vi "UAS_Ground_Station_v1.02.vi"() -> ()   [LabVIEW 2020]
uses:
  <vilib>/Utility/miscctls.llb/LVForegroundBackgroundColorsTypeDef.ctl
  76567d80-d4f7-4105-a57e-45636684cd43.vi
  66f1963f-959d-441b-b800-4ec726fb55a9.vi
  2b59091c-cbc3-4e12-b608-60c3f7d5f04d.vi
  4d25b74f-ab1f-40a0-8ca1-83bd5f887b88.vi
panel:
  out "EXCEL_STATUS":string
  in  "Export":bool
  out "TimeoutCount":dbl
  out "TotalLatencyArray":dbl[](array[numeric])
  in  "Total Latency":bool
  out "Stop_buf":bool=TRUE
  in  "Rx Latency":bool
  out "RxSampleArray":dbl[](array[numeric])
  out "RxLatencyArray":dbl[](array[numeric])
  out "Rx Timer Start":dbl
  out "Latency Data":cluster{"Value":i32[], "Value":u32[]}[](graph)
  in  "Tx Latency":bool
  out "TxSampleArray":dbl[](array[numeric])
  out "TxLatencyArray":u32[](array[numeric])
  out "Rx_Index":dbl
  out "Tx_Index":dbl
  out "Tx Timer Start":u32
  in  "Tx Data":T1 {"Position(X):" format="%_6g"; "Position(Y):" format="%_6g"; "Position(Z):" format="%_6g"; "Rotation(X):" format="%_6g"; "Rotation(Y):" format="%_6g"; "Rotation(Z):" format="%_6g"; "Mode:" format="%#.6f"}
  out "Rx Data":T2
  out "number":i32
  out "Rx Struct Data":dbl[](array[numeric])
  out "Rx array":string[](array[string])
  out "Index":dbl
  out "stringBuffer":string
  out "Rx Status":bool
  out "Tx Status":bool
  in  "OK Button":bool
  out "IP":string
  out "Rx String":string
  out "Tx String":string
  in  "Rx Port":string="3000"
  in  "Tx Port":string="2390"
  in  "Address":string="192.168.1.244"
  in  "stop":bool
  # "UAS Ground Station Control"
  # "UAS UDP Latency Data"
  # "Network Configuration"
  # "Rx Data"
  # "Tx Data"
  # "Communication Controls"
  # "Status Indicators"
  # "Plot Contols"
  # "Rx"
  # "Tx"
  # "Total"
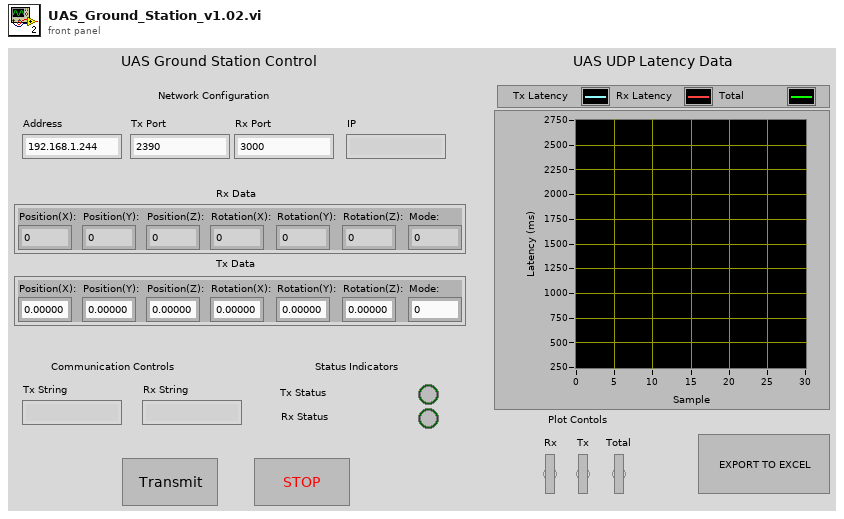
[diagram p1: front panel]
types:
  T1 = cluster{"Mode:":i32, "Rotation(Z):":dbl, "Rotation(Y):":dbl, "Rotation(X):":dbl, "Position(Z):":dbl, "Position(Y):":dbl, "Position(X):":dbl}
  T2 = cluster{"Position(X):":dbl, "Position(Y):":dbl, "Position(Z):":dbl, "Rotation(X):":dbl, "Rotation(Y):":dbl, "Rotation(Z):":dbl, "Mode:":i32}
  T3 = enum8{"Enabled", "Disabled", "Disabled and Grayed Out"}
  T4 = typedef "LVForegroundBackgroundColorsTypeDef.ctl" = cluster{"Foreground Color":u32, "Background Color":u32}
  T5 = cluster{"Value[0]":dbl, "Value[1]":dbl, "Value[2]":dbl, "Value[3]":dbl, "Value[4]":dbl, "Value[5]":dbl}
  T6 = cluster{"Value[0]":dbl, "Value[1]":dbl, "Value[2]":dbl, "Value[3]":dbl, "Value[4]":dbl, "Value[5]":dbl, "Value":i32}
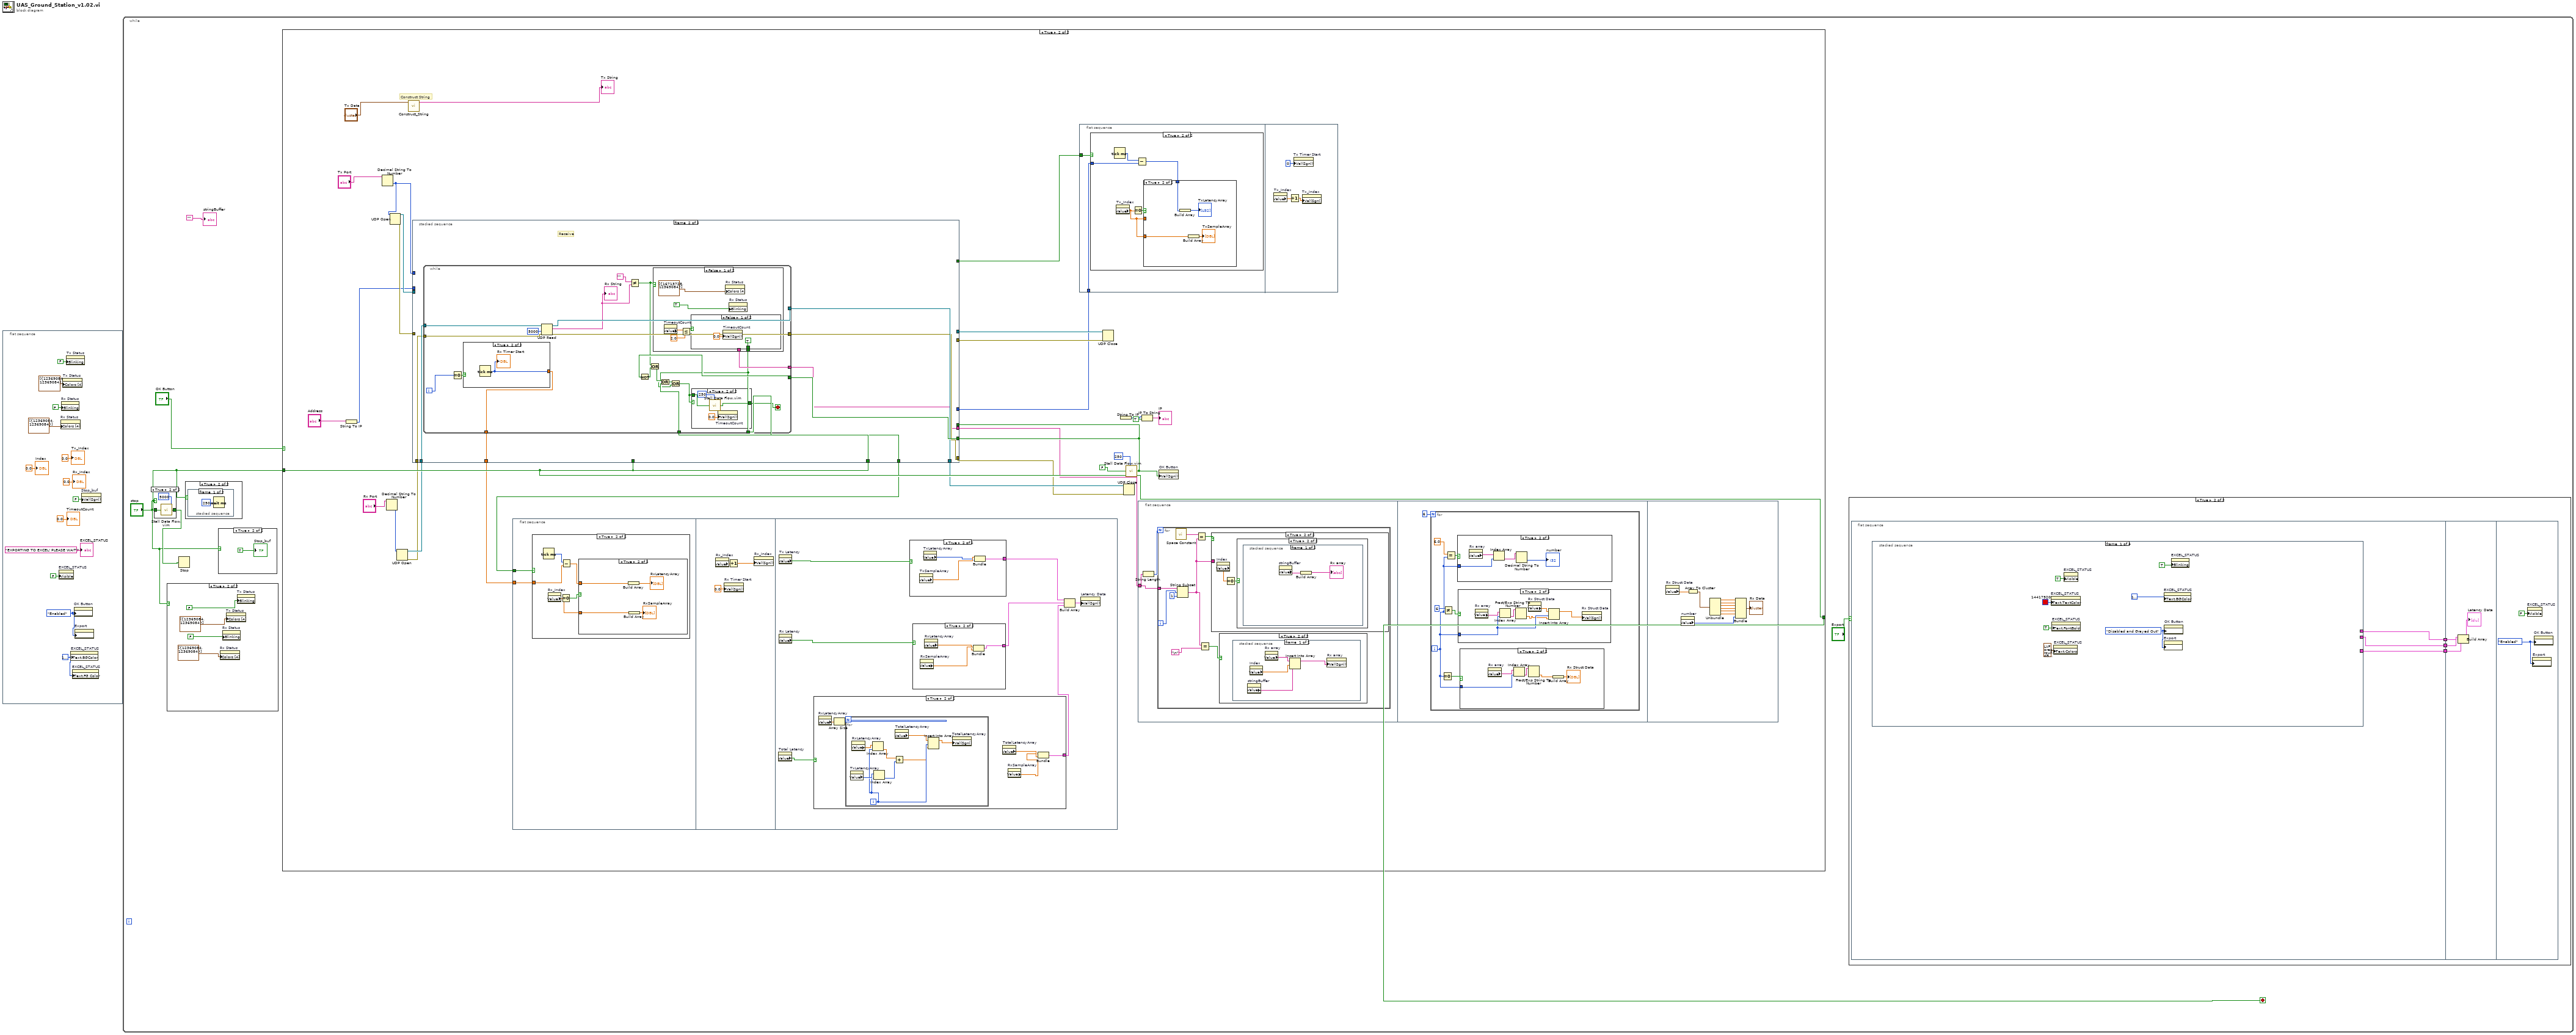
[diagram p0: block diagram]
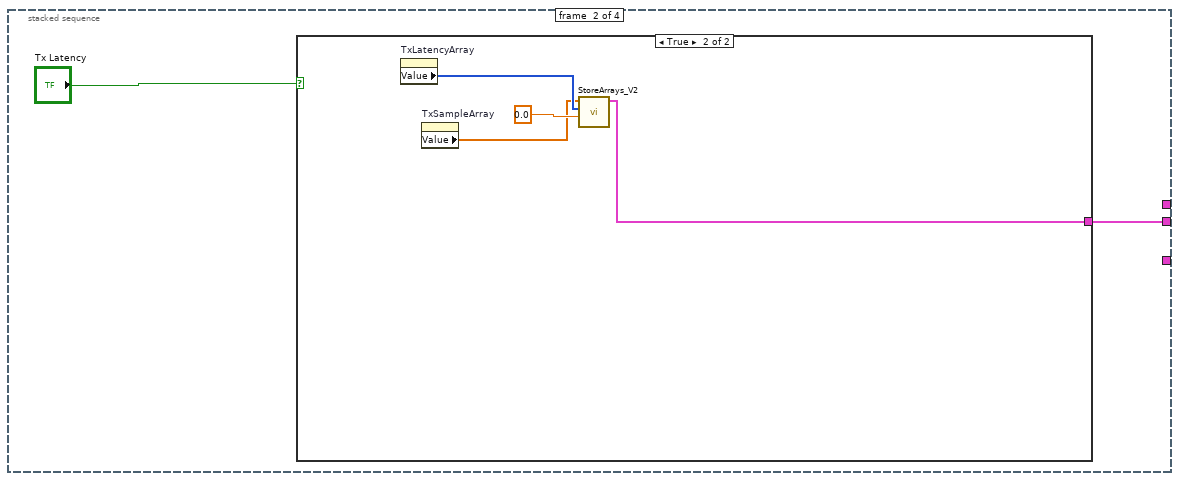
[diagram p5: hidden frame]
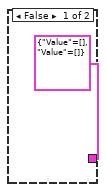
[diagram p6: hidden frame]
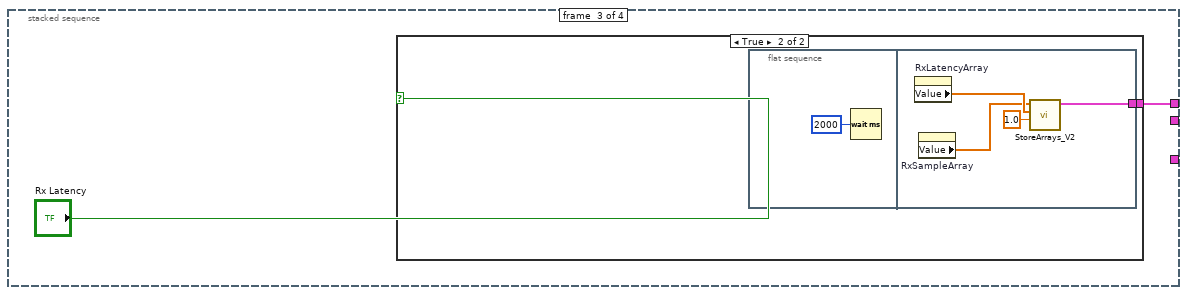
[diagram p7: hidden frame]
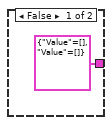
[diagram p8: hidden frame]
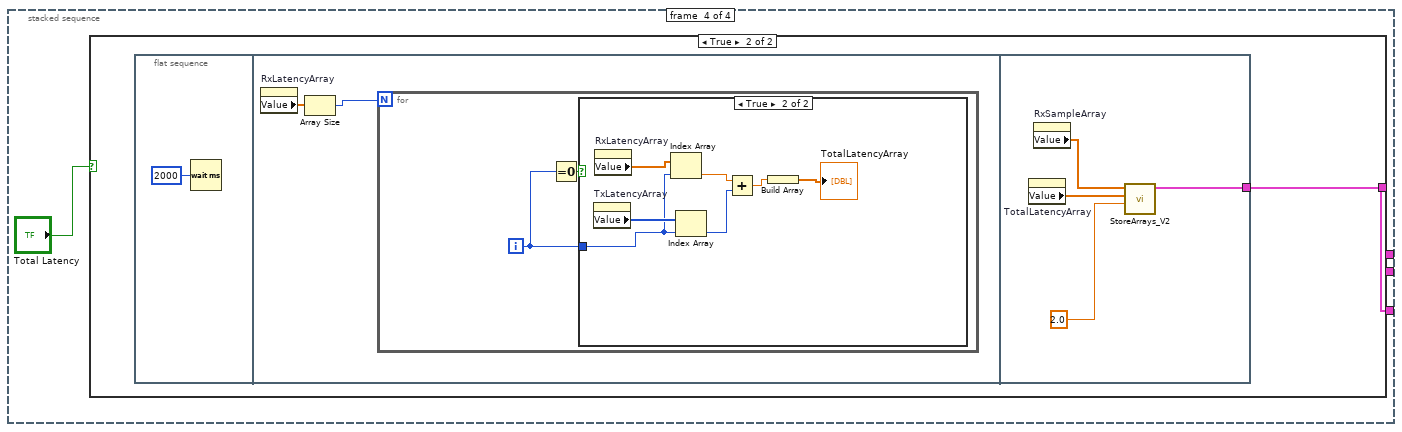
[diagram p9: hidden frame]
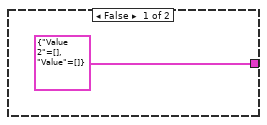
[diagram p10: hidden frame]
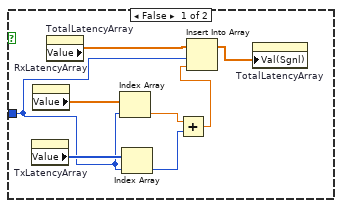
[diagram p11: hidden frame]
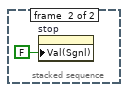
[diagram p14: hidden frame]
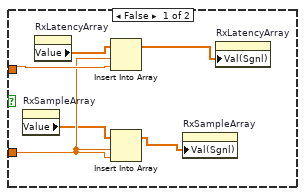
[diagram p17: hidden frame]
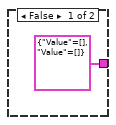
[diagram p18: hidden frame]
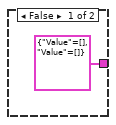
[diagram p19: hidden frame]
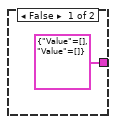
[diagram p20: hidden frame]
diagram:
  n1 = flat-sequence {
    frame #0 {
      w1 = u32 16777216 ("Text.Text Colors:BG Color")
      w2 = T3."Enabled" ("Disabled")
      n2 = property on="EXCEL_STATUS" class="Str"("Visible"=FALSE) -> ()  [unwired: 2 in, 2 out]
      n3 = property on="Rx Status" class="Bool (strict)"("Colors [4]"=cluster{u32, u32}[] [{12369084, 12369084}]) -> ()  [unwired: 2 in, 2 out]
      n4 = property on="Rx Status" class="Bool (strict)"("Blinking"=FALSE) -> ()  [unwired: 2 in, 2 out]
      n5 = property on="Tx Status" class="Bool (strict)"("Colors [4]"=cluster{u32, u32}[] [{12369084, 12369084}]) -> ()  [unwired: 2 in, 2 out]
      n6 = property on="Tx Status" class="Bool (strict)"("Blinking"=FALSE) -> ()  [unwired: 2 in, 2 out]
      n7 = property on="EXCEL_STATUS" class="Str"("Text.BGColor"=w1) -> ()  [unwired: 2 in, 2 out]
      n8 = property on="EXCEL_STATUS" class="Str"("Text.FG Color"=w1) -> ()  [unwired: 2 in, 2 out]
      n9 = property on="OK Button" class="Bool (strict)"("DisabledEnum"=w2) -> ()  [unwired: 2 in, 2 out]
      n10 = property on="Export" class="Bool"("DisabledEnum"=w2) -> ()  [unwired: 2 in, 2 out]
      n11 = property on="Stop_buf" class="Bool (strict)"("Val(Sgnl)"=FALSE ("Value (Signaling)")) -> ()  [unwired: 2 in, 2 out]
      "Index" <- 0.0 ("Index")
      "Tx_Index" <- 0.0 ("Tx_Index")
      "Rx_Index" <- 0.0 ("Rx_Index")
      "TimeoutCount" <- 0.0 ("TimeoutCount")
      "EXCEL_STATUS" <- "EXPORTING TO EXCEL! PLEASE WAIT!" ("String")
    }
  }
  n12 = while {
    stop <- w15 stop-if-true
    n13 = case shown="True" "stop" {
      tunnel: [w21 w23] -> w18
      tunnel: "stop" -> [w21 w22]
      frame False {
      }
      frame True {
        n14 = call "Stall Data Flow.vim"("value in"=w22, "milliseconds to wait"=u32 5000 ("millisecond timer value")) -> ("value out"=w23:bool)  [unwired: 1 out]
      }
    }
    n15 = case shown="True" "stop" {
      frame False {
      }
      frame True {
        n16 = property on="Rx Status" class="Bool (strict)"("Colors [4]"=cluster{u32, u32}[] [{12369084, 12369084}]) -> ()  [unwired: 2 in, 2 out]
        n17 = property on="Rx Status" class="Bool (strict)"("Blinking"=FALSE) -> ()  [unwired: 2 in, 2 out]
        n18 = property on="Tx Status" class="Bool (strict)"("Colors [4]"=cluster{u32, u32}[] [{12369084, 12369084}]) -> ()  [unwired: 2 in, 2 out]
        n19 = property on="Tx Status" class="Bool (strict)"("Blinking"=FALSE) -> ()  [unwired: 2 in, 2 out]
      }
    }
    n20 = Stop(stop? (T)=w18) -> ()
    n21 = case shown="True" "stop" {
      frame False {
      }
      frame True {
        n22 = stacked-sequence {
          frame #0 {
            n23 = Wait (ms)(milliseconds to wait=u32 250) -> ()  [unwired: 1 out]
          }
          frame #1 {
            n24 = property on="stop" class="Bool (strict)"("Val(Sgnl)"=FALSE ("Value (Signaling)")) -> ()  [unwired: 2 in, 2 out]
          }
        }
      }
    }
    n25 = case shown="True" "stop" {
      frame False {
      }
      frame True {
        "Stop_buf" <- TRUE
      }
    }
    n26 = case shown="True" "OK Button" {
      tunnel: [_ w102] -> w15
      tunnel: "stop" -> [_ w102]
      frame False {
      }
      frame True {
        # "Construct String"
        n27 = String To IP(1:"Address") -> (0:w111:u32)
        n28 = Decimal String To Number(string="Tx Port") -> (number=w109:i32)  [unwired: 2 in, 1 out]
        n29 = Decimal String To Number(string="Rx Port") -> (number=w116:i32)  [unwired: 2 in, 1 out]
        n30 = UDP Open(11:w109) -> (port=w121:refnum<k16>, 0:w120:errorcluster)  [unwired: 4 in, 1 out]
        n31 = UDP Open(11:w116) -> (port=w101:refnum<k16>, 0:w100:errorcluster)  [unwired: 4 in, 1 out]
        n32 = call "Construct_String.vi"("Tx Data"="Tx Data") -> ("String"=→"Tx String":string)  [unwired: 10 in]
        n33 = flat-sequence {
          tunnel: w95 -> [w123]
          tunnel: w94 -> [w122]
          frame #0 {
            n34 = case shown="True" w123 {
              tunnel: w122 -> [_ w127]
              frame False {
              }
              frame True {
                n35 = Tick Count (ms)() -> (millisecond timer value=w128:u32)
                n36 = property on="Rx_Index" class="DigNum (strict)"() -> ("Value"=w124:dbl)  [unwired: 2 in, 2 out]
                n37 = Equal To 0?(x=w124) -> (x = 0?=w126:bool)
                n38 = Subtract(x=w128, y=w127) -> (x-y=w125:dbl)
                n39 = case shown="True" w126 {
                  tunnel: w125 -> [w132 w138]
                  tunnel: w124 -> [w131 w136]
                  frame False {
                    n40 = property on="RxSampleArray" class="Arr (strict)"() -> ("Value"=w130:dbl[])  [unwired: 2 in, 2 out]
                    n41 = property on="RxLatencyArray" class="Arr (strict)"() -> ("Value"=w134:dbl[])  [unwired: 2 in, 2 out]
                    n42 = Insert Into Array(array=w134, index=w131, new element=w132) -> (w133:dbl[])
                    n43 = Insert Into Array(array=w130, index=w131, new element=w131) -> (w129:dbl[])
                    n44 = property on="RxSampleArray" class="Arr (strict)"("Val(Sgnl)"=w129) -> ()  [unwired: 2 in, 2 out]
                    n45 = property on="RxLatencyArray" class="Arr (strict)"("Val(Sgnl)"=w133) -> ()  [unwired: 2 in, 2 out]
                  }
                  frame True {
                    n46 = Build Array(w138) -> (→"RxLatencyArray":dbl[])
                    n47 = Build Array(w136) -> (→"RxSampleArray":dbl[])
                  }
                }
              }
            }
          }
          frame #1 {
            n48 = property on="Rx_Index" class="DigNum (strict)"() -> ("Value"=w141:dbl)  [unwired: 2 in, 2 out]
            n49 = property on="Rx Timer Start" class="DigNum (strict)"("Val(Sgnl)"=0.0 ("Value (Signaling)")) -> ()  [unwired: 2 in, 2 out]
            n50 = Increment(x=w141) -> (x+1=w140:dbl)
            n51 = property on="Rx_Index" class="DigNum (strict)"("Val(Sgnl)"=w140) -> ()  [unwired: 2 in, 2 out]
          }
          frame #2 {
            n52 = property on="Total Latency" class="Bool (strict)"() -> ("Value"=w148:bool)  [unwired: 2 in, 2 out]
            n53 = property on="Tx Latency" class="Bool (strict)"() -> ("Value"=w146:bool)  [unwired: 2 in, 2 out]
            n54 = property on="Rx Latency" class="Bool (strict)"() -> ("Value"=w147:bool)  [unwired: 2 in, 2 out]
            n55 = case shown="True" w148 {
              tunnel: [cluster{"Value":dbl[], "Value":dbl[]} {"Value"=[], "Value"=[]} w152] -> w143
              frame False {
              }
              frame True {
                n56 = property on="RxLatencyArray" class="Arr (strict)"() -> ("Value"=w154:dbl[])  [unwired: 2 in, 2 out]
                n57 = Array Size(array=w154) -> (size(s)=w153:i32)
                n58 = for {
                  N: w153 -> [_]
                  i -> [w158]
                  n59 = property on="TxLatencyArray" class="Arr (strict)"() -> ("Value"=w159:u32[])  [unwired: 2 in, 2 out]
                  n60 = property on="RxLatencyArray" class="Arr (strict)"() -> ("Value"=w160:dbl[])  [unwired: 2 in, 2 out]
                  n61 = Index Array(array=w160, index=w158) -> (element=w157:dbl)
                  n62 = Index Array(array=w159, index=w158) -> (element=w156:u32)
                  n63 = Add(x=w157, y=w156) -> (x+y=w155:dbl)
                  n64 = property on="TotalLatencyArray" class="Arr (strict)"() -> ("Value"=w161:dbl[])  [unwired: 2 in, 2 out]
                  n65 = Insert Into Array(array=w161, index=w158, new element=w155) -> (w162:dbl[])
                  n66 = property on="TotalLatencyArray" class="Arr (strict)"("Val(Sgnl)"=w162) -> ()  [unwired: 2 in, 2 out]
                }
                n67 = property on="TotalLatencyArray" class="Arr (strict)"() -> ("Value"=w151:dbl[])  [unwired: 2 in, 2 out]
                n68 = property on="RxSampleArray" class="Arr (strict)"() -> ("Value"=w150:dbl[])  [unwired: 2 in, 2 out]
                n69 = Bundle("Value"=w150, "Value"=w151) -> (w152:cluster{"Value":dbl[], "Value":dbl[]})  [unwired: 1 in]
              }
            }
            n70 = case shown="True" w146 {
              tunnel: [cluster{"Value":u32[], "Value":dbl[]} {"Value"=[], "Value"=[]} w170] -> w145
              frame False {
              }
              frame True {
                n71 = property on="TxSampleArray" class="Arr (strict)"() -> ("Value"=w169:dbl[])  [unwired: 2 in, 2 out]
                n72 = property on="TxLatencyArray" class="Arr (strict)"() -> ("Value"=w168:u32[])  [unwired: 2 in, 2 out]
                n73 = Bundle("Value"=w169, "Value"=w168) -> (w170:cluster{"Value":dbl[], "Value":u32[]})  [unwired: 1 in]
              }
            }
            n74 = case shown="True" w147 {
              tunnel: [cluster{"Value":dbl[], "Value":dbl[]} {"Value"=[], "Value"=[]} w166] -> w144
              frame False {
              }
              frame True {
                n75 = property on="RxSampleArray" class="Arr (strict)"() -> ("Value"=w165:dbl[])  [unwired: 2 in, 2 out]
                n76 = property on="RxLatencyArray" class="Arr (strict)"() -> ("Value"=w164:dbl[])  [unwired: 2 in, 2 out]
                n77 = Bundle("Value"=w165, "Value"=w164) -> (w166:cluster{"Value":dbl[], "Value":dbl[]})  [unwired: 1 in]
              }
            }
            n78 = Build Array(w145, w144, w143) -> (w142:cluster{"Value":dbl[], "Value":dbl[]}[])
            n79 = property on="Latency Data" class="XYGraph (strict)"("Val(Sgnl)"=w142) -> ()  [unwired: 2 in, 2 out]
          }
        }
        n80 = flat-sequence {
          tunnel: w104 -> [w300]
          tunnel: w103 -> [w299]
          frame #0 {
            n81 = case shown="True" w300 {
              tunnel: w299 -> [_ w305]
              frame False {
              }
              frame True {
                n82 = Tick Count (ms)() -> (millisecond timer value=w304:u32)
                n83 = property on="Tx_Index" class="DigNum (strict)"() -> ("Value"=w301:dbl)  [unwired: 2 in, 2 out]
                n84 = Equal To 0?(x=w301) -> (x = 0?=w303:bool)
                n85 = Subtract(x=w304, y=w305) -> (x-y=w302:u32)
                n86 = case shown="True" w303 {
                  tunnel: w302 -> [w309 w316]
                  tunnel: w301 -> [w310 _]
                  tunnel: w301 -> [w307 w314]
                  frame False {
                    n87 = property on="TxLatencyArray" class="Arr (strict)"() -> ("Value"=w311:u32[])  [unwired: 2 in, 2 out]
                    n88 = property on="TxSampleArray" class="Arr (strict)"() -> ("Value"=w308:dbl[])  [unwired: 2 in, 2 out]
                    n89 = Insert Into Array(array=w311, index=w310, new element=w309) -> (w312:u32[])
                    n90 = Insert Into Array(array=w308, index=w307, new element=w307) -> (w306:dbl[])
                    n91 = property on="TxLatencyArray" class="Arr (strict)"("Val(Sgnl)"=w312) -> ()  [unwired: 2 in, 2 out]
                    n92 = property on="TxSampleArray" class="Arr (strict)"("Val(Sgnl)"=w306) -> ()  [unwired: 2 in, 2 out]
                  }
                  frame True {
                    n93 = Build Array(w316) -> (→"TxLatencyArray":u32[])
                    n94 = Build Array(w314) -> (→"TxSampleArray":dbl[])
                  }
                }
              }
            }
          }
          frame #1 {
            n95 = property on="Tx_Index" class="DigNum (strict)"() -> ("Value"=w318:dbl)  [unwired: 2 in, 2 out]
            n96 = Increment(x=w318) -> (x+1=w317:dbl)
            n97 = property on="Tx Timer Start" class="DigNum (strict)"("Val(Sgnl)"=u32 0 ("Value (Signaling)")) -> ()  [unwired: 2 in, 2 out]
            n98 = property on="Tx_Index" class="DigNum (strict)"("Val(Sgnl)"=w317) -> ()  [unwired: 2 in, 2 out]
          }
        }
        n99 = String To IP() -> (0:w115:u32)  [unwired: 1 in]
        n100 = call "Stall Data Flow.vim"("value in"=FALSE, "milliseconds to wait"=u32 250) -> ("value out"=w99:bool)  [unwired: 1 out]
        n101 = stacked-sequence {
          tunnel: w121 -> [w180 _]
          tunnel: w120 -> [w179 _]
          tunnel: [w178 _] -> w119
          tunnel: [w177 _] -> w118
          tunnel: w111 -> [w176 _]
          tunnel: w109 -> [w175 _]
          tunnel: w99 -> [w174 _]
          tunnel: w102 -> [w173 _]
          tunnel: [w172 _] -> w104
          tunnel: [w171 _] -> w103
          tunnel: w102 -> [_ w254]
          tunnel: w101 -> [_ w253]
          tunnel: w100 -> [_ w252]
          tunnel: w99 -> [_ w251]
          tunnel: [_ w250] -> w98
          tunnel: [_ w249] -> w97
          tunnel: [_ w248] -> w96
          tunnel: [_ w247] -> w95
          tunnel: [_ w246] -> w94
          frame #0 {
            # "Transmit"
            n102 = while {
              tunnel: w180 -> [w197]
              tunnel: w179 -> [w196]
              tunnel: [w190] -> w178
              tunnel: [w189] -> w177
              tunnel: w175 -> [w195]
              tunnel: w176 -> [w194]
              tunnel: w173 -> [w193]
              tunnel: w174 -> [w192]
              tunnel: [w181] -> w172
              tunnel: [w185] -> w171
              i -> [w183]
              stop <- w188 stop-if-true
              n103 = Equal To 0?(x=w183) -> (x = 0?=w184:bool)
              n104 = property on="Tx String" class="Str"() -> ("Value"=w186:string)  [unwired: 2 in, 2 out]
              n105 = case shown="True" w184 {
                tunnel: [w198 w199] -> w185
                frame False {
                  n106 = property on="Tx Timer Start" class="DigNum (strict)"() -> ("Value"=w198:u32)  [unwired: 2 in, 2 out]
                }
                frame True {
                  n107 = Tick Count (ms)() -> (millisecond timer value=w199:u32)
                  "Tx Timer Start" <- w199
                }
              }
              n108 = Not(x=w192) -> (.not. x?=w191:bool)
              n109 = Or(x=w191, y=w193) -> (x .or. y?=w188:bool)
              n110 = while {
                tunnel: w186 -> [w226]
                tunnel: w195 -> [w225]
                tunnel: w194 -> [w224]
                shift-right: [w221] -> w190
                shift-left: w197 -> [w228]
                shift-right: [w220] -> w189
                shift-left: w196 -> [w227]
                tunnel: w188 -> [w217]
                tunnel: [w216] -> w187
                tunnel: [w212] -> w182
                stop <- w214 stop-if-true
                n111 = UDP Write(address=w224, port or service name=w225, connection ID=w228, data in=w226, 8:w227) -> (error out=w222:errorcluster, 3:w223:refnum<k16>)  [unwired: 1 in]
                n112 = UDP Read(connection ID=w223, timeout ms (25000)=5000, 8:w222) -> (data out=w219:string, error out=w220:errorcluster, 3:w221:refnum<k16>)  [unwired: 1 in, 2 out]
                n113 = Equal?(x="OK", y=w219) -> (x = y?=w216:bool)
                n114 = case shown="False" w216 {
                  tunnel: [w235 TRUE] -> w215
                  tunnel: [w234 FALSE] -> w212
                  frame False {
                    n115 = property on="TimeoutCount" class="DigNum (strict)"() -> ("Value"=w237:dbl)  [unwired: 2 in, 2 out]
                    n116 = Wait (ms)(milliseconds to wait=u32 250) -> ()  [unwired: 1 out]
                    n117 = Less Or Equal?(x=w237, y=2.0) -> (x <= y?=w234:bool)
                    n118 = case shown="False" w234 {
                      tunnel: [TRUE FALSE] -> w235
                      frame False {
                        n119 = property on="TimeoutCount" class="DigNum (strict)"("Val(Sgnl)"=0.0 ("Value (Signaling)")) -> ()  [unwired: 2 in, 2 out]
                      }
                      frame True {
                        n120 = property on="TimeoutCount" class="DigNum (strict)"() -> ("Value"=w243:dbl)  [unwired: 2 in, 2 out]
                        n121 = Increment(x=w243) -> (x+1=w242:dbl)
                        n122 = property on="TimeoutCount" class="DigNum (strict)"("Val(Sgnl)"=w242) -> ()  [unwired: 2 in, 2 out]
                      }
                    }
                  }
                  frame True {
                  }
                }
                n123 = Or(x=w215, y=w217) -> (x .or. y?=w213:bool)
                n124 = case shown="True" w213 {
                  tunnel: [w229 w232] -> w214
                  tunnel: w213 -> [w229 w233]
                  frame False {
                  }
                  frame True {
                    n125 = call "Stall Data Flow.vim"("value in"=w233, "milliseconds to wait"=u32 250) -> ("value out"=w232:bool)  [unwired: 1 out]
                    n126 = property on="TimeoutCount" class="DigNum (strict)"("Val(Sgnl)"=0.0 ("Value (Signaling)")) -> ()  [unwired: 2 in, 2 out]
                  }
                }
              }
              n127 = case shown="True" w187 {
                tunnel: w182 -> [w201 _]
                tunnel: [w200 TRUE] -> w181
                frame False {
                  n128 = property on="Tx Status" class="Bool (strict)"("Colors [4]"=cluster{u32, u32}[] [{16713728, 12369084}]) -> ()  [unwired: 2 in, 2 out]
                  n129 = property on="Tx Status" class="Bool (strict)"("Blinking"=TRUE) -> ()  [unwired: 2 in, 2 out]
                  n130 = case shown="False" w201 {
                    tunnel: [TRUE FALSE] -> w200
                    frame False {
                    }
                    frame True {
                    }
                  }
                }
                frame True {
                  n131 = property on="Tx Status" class="Bool (strict)"("Colors [4]"=cluster{u32, u32}[] [{46091, 12369084}]) -> (error out=w208:errorcluster)  [unwired: 2 in, 1 out]
                  n132 = property on="Tx Status" class="Bool (strict)"(error in=w208, "Blinking"=FALSE) -> ()  [unwired: 1 in, 2 out]
                  "Tx Status" <- TRUE
                }
              }
            }
          }
          frame #1 {
            # "Receive"
            n133 = while {
              tunnel: w254 -> [w270]
              tunnel: w253 -> [w274]
              tunnel: w252 -> [w273]
              tunnel: [w272] -> w250
              tunnel: [w271] -> w249
              tunnel: w251 -> [w269]
              tunnel: [w263] -> w248
              tunnel: [w258] -> w247
              tunnel: [w260] -> w246
              i -> [w261]
              stop <- w257 stop-if-true
              n134 = Equal To 0?(x=w261) -> (x = 0?=w262:bool)
              n135 = case shown="True" w262 {
                tunnel: [w280 w281] -> w260
                frame False {
                  n136 = property on="Rx Timer Start" class="DigNum (strict)"() -> ("Value"=w280:dbl)  [unwired: 2 in, 2 out]
                }
                frame True {
                  n137 = Tick Count (ms)() -> (millisecond timer value=w281:u32)
                  "Rx Timer Start" <- w281
                }
              }
              n138 = UDP Read(connection ID=w274, timeout ms (25000)=5000, 8:w273) -> (data out=w267:string, error out=w271:errorcluster, 3:w272:refnum<k16>)  [unwired: 1 in, 2 out]
              "Rx String" <- w267
              n139 = Not Equal?(x="", y=w267) -> (x != y?=w264:bool)
              n140 = Not(x=w269) -> (.not. x?=w266:bool)
              n141 = Or(x=w264, y=w266) -> (x .or. y?=w265:bool)
              n142 = case shown="False" w264 {
                tunnel: [_ w295] -> w263
                tunnel: [w285 TRUE] -> w258
                frame False {
                  n143 = property on="TimeoutCount" class="DigNum (strict)"() -> ("Value"=w284:dbl)  [unwired: 2 in, 2 out]
                  n144 = Less Or Equal?(x=w284, y=2.0) -> (x <= y?=w282:bool)
                  n145 = case shown="False" w282 {
                    tunnel: [TRUE FALSE] -> w285
                    frame False {
                      n146 = property on="TimeoutCount" class="DigNum (strict)"("Val(Sgnl)"=0.0 ("Value (Signaling)")) -> ()  [unwired: 2 in, 2 out]
                    }
                    frame True {
                      n147 = property on="TimeoutCount" class="DigNum (strict)"() -> ("Value"=w291:dbl)  [unwired: 2 in, 2 out]
                      n148 = Increment(x=w291) -> (x+1=w290:dbl)
                      n149 = property on="TimeoutCount" class="DigNum (strict)"("Val(Sgnl)"=w290) -> ()  [unwired: 2 in, 2 out]
                      n150 = Wait (ms)(milliseconds to wait=u32 250) -> ()  [unwired: 1 out]
                    }
                  }
                  n151 = property on="Rx Status" class="Bool (strict)"("Colors [4]"=cluster{u32, u32}[] [{16713728, 12369084}]) -> ()  [unwired: 2 in, 2 out]
                  n152 = property on="Rx Status" class="Bool (strict)"("Blinking"=TRUE) -> ()  [unwired: 2 in, 2 out]
                }
                frame True {
                  n153 = property on="Rx String" class="Str"() -> ("Value"=w295:string)  [unwired: 2 in, 2 out]
                  n154 = property on="Rx Status" class="Bool (strict)"("Blinking"=FALSE) -> ()  [unwired: 2 in, 2 out]
                  n155 = property on="Rx Status" class="Bool (strict)"("Colors [4]"=cluster{u32, u32}[] [{46091, 12369084}]) -> ()  [unwired: 2 in, 2 out]
                  "Rx Status" <- TRUE
                }
              }
              n156 = Or(x=w265, y=w270) -> (x .or. y?=w259:bool)
              n157 = Or(x=w259, y=w258) -> (x .or. y?=w256:bool)
              n158 = case shown="True" w256 {
                tunnel: [w275 w278] -> w257
                tunnel: w256 -> [w275 w279]
                frame False {
                }
                frame True {
                  n159 = call "Stall Data Flow.vim"("value in"=w279, "milliseconds to wait"=u32 250) -> ("value out"=w278:bool)  [unwired: 1 out]
                  n160 = property on="TimeoutCount" class="DigNum (strict)"("Val(Sgnl)"=0.0 ("Value (Signaling)")) -> ()  [unwired: 2 in, 2 out]
                }
              }
            }
          }
        }
        n161 = UDP Close(connection ID=w119, 8:w118) -> ()  [unwired: 2 out]
        n162 = UDP Close(connection ID=w98, 8:w97) -> ()  [unwired: 2 out]
        n163 = flat-sequence {
          tunnel: w96 -> [w320]
          frame #0 {
            n164 = String Length(string=w320) -> (length=w321:i32)
            n165 = for {
              N: w321 -> [_]
              tunnel: w320 -> [w329]
              i -> [w327]
              n166 = call <vilib>:"Space Constant.vi"() -> ("String"=w325:string)
              n167 = String Subset(string=w329, offset (0)=w327, length (rest)=1 ("length (rest)")) -> (substring=w324:string)
              n168 = Equal?(x=w325, y=w324) -> (x = y?=w326:bool)
              n169 = Equal?(x=w324, y="\n") -> (x = y?=w323:bool)
              n170 = case shown="True" w326 {
                tunnel: w324 -> [w336 _]
                frame False {
                  n171 = property on="stringBuffer" class="Str"() -> ("Value"=w338:string)  [unwired: 2 in, 2 out]
                  n172 = Concatenate Strings(w338, w336) -> (w337:string)
                  n173 = property on="stringBuffer" class="Str"("Val(Sgnl)"=w337) -> ()  [unwired: 2 in, 2 out]
                }
                frame True {
                  n174 = property on="Index" class="DigNum (strict)"() -> ("Value"=w339:dbl)  [unwired: 2 in, 2 out]
                  n175 = Equal To 0?(x=w339) -> (x = 0?=w340:bool)
                  n176 = case shown="True" w340 {
                    frame False {
                      n177 = stacked-sequence {
                        frame #0 {
                          n178 = property on="Index" class="DigNum (strict)"() -> ("Value"=w344:dbl)  [unwired: 2 in, 2 out]
                          n179 = property on="Rx array" class="Arr (strict)"() -> ("Value"=w343:string[])  [unwired: 2 in, 2 out]
                          n180 = property on="stringBuffer" class="Str"() -> ("Value"=w342:string)  [unwired: 2 in, 2 out]
                          n181 = Insert Into Array(array=w343, index=w344, new element=w342) -> (w341:string[])
                          n182 = property on="Rx array" class="Arr (strict)"("Val(Sgnl)"=w341) -> ()  [unwired: 2 in, 2 out]
                        }
                        frame #1 {
                          n183 = property on="Index" class="DigNum (strict)"() -> ("Value"=w347:dbl)  [unwired: 2 in, 2 out]
                          n184 = Increment(x=w347) -> (x+1=w346:dbl)
                          n185 = property on="Index" class="DigNum (strict)"("Val(Sgnl)"=w346) -> ()  [unwired: 2 in, 2 out]
                          n186 = property on="stringBuffer" class="Str"("Val(Sgnl)"="") -> ()  [unwired: 2 in, 2 out]
                        }
                      }
                    }
                    frame True {
                      n187 = stacked-sequence {
                        frame #0 {
                          n188 = property on="stringBuffer" class="Str"() -> ("Value"=w349:string)  [unwired: 2 in, 2 out]
                          n189 = Build Array(w349) -> (→"Rx array":string[])
                        }
                        frame #1 {
                          n190 = property on="Index" class="DigNum (strict)"() -> ("Value"=w351:dbl)  [unwired: 2 in, 2 out]
                          n191 = Increment(x=w351) -> (x+1=w350:dbl)
                          n192 = property on="stringBuffer" class="Str"("Val(Sgnl)"="") -> ()  [unwired: 2 in, 2 out]
                          n193 = property on="Index" class="DigNum (strict)"("Val(Sgnl)"=w350) -> ()  [unwired: 2 in, 2 out]
                        }
                      }
                    }
                  }
                }
              }
              n194 = case shown="True" w323 {
                frame False {
                }
                frame True {
                  n195 = stacked-sequence {
                    frame #0 {
                      n196 = property on="stringBuffer" class="Str"() -> ("Value"=w330:string)  [unwired: 2 in, 2 out]
                      n197 = property on="Index" class="DigNum (strict)"() -> ("Value"=w331:dbl)  [unwired: 2 in, 2 out]
                      n198 = property on="Rx array" class="Arr (strict)"() -> ("Value"=w332:string[])  [unwired: 2 in, 2 out]
                      n199 = Insert Into Array(array=w332, index=w331, new element=w330) -> (w333:string[])
                      n200 = property on="Rx array" class="Arr (strict)"("Val(Sgnl)"=w333) -> ()  [unwired: 2 in, 2 out]
                    }
                    frame #1 {
                      n201 = property on="stringBuffer" class="Str"("Val(Sgnl)"="") -> ()  [unwired: 2 in, 2 out]
                      n202 = property on="Index" class="DigNum (strict)"("Val(Sgnl)"=0.0 ("Value (Signaling)")) -> ()  [unwired: 2 in, 2 out]
                    }
                  }
                }
              }
            }
          }
          frame #1 {
            n203 = for {
              N: 6 -> [_]
              i -> [w354]
              n204 = Equal To 0?(x=w354) -> (x = 0?=w357:bool)
              n205 = Not Equal?(x=6, y=w354) -> (x != y?=w358:bool)
              n206 = Equal?(x=6.0, y=w354) -> (x = y?=w356:bool)
              n207 = case shown="True" w356 {
                tunnel: w354 -> [_ w362]
                frame False {
                }
                frame True {
                  n208 = property on="Rx array" class="Arr (strict)"() -> ("Value"=w363:string[])  [unwired: 2 in, 2 out]
                  n209 = Index Array(array=w363, index=w362) -> (element=w361:string)
                  n210 = Decimal String To Number(string=w361) -> (number=→"number":i32)  [unwired: 2 in, 1 out]
                }
              }
              n211 = case shown="True" w358 {
                tunnel: w354 -> [_ w373]
                frame False {
                }
                frame True {
                  n212 = property on="Rx array" class="Arr (strict)"() -> ("Value"=w374:string[])  [unwired: 2 in, 2 out]
                  n213 = Index Array(array=w374, index=w373) -> (element=w372:string)
                  n214 = Fract/Exp String To Number(string=w372) -> (number=w371:dbl)  [unwired: 3 in, 1 out]
                  n215 = property on="Rx Struct Data" class="Arr (strict)"() -> ("Value"=w369:dbl[])  [unwired: 2 in, 2 out]
                  n216 = Insert Into Array(array=w369, index=w373, new element=w371) -> (w370:dbl[])
                  n217 = property on="Rx Struct Data" class="Arr (strict)"("Val(Sgnl)"=w370) -> ()  [unwired: 2 in, 2 out]
                }
              }
              n218 = case shown="True" w357 {
                tunnel: w354 -> [_ w367]
                frame False {
                }
                frame True {
                  n219 = property on="Rx array" class="Arr (strict)"() -> ("Value"=w368:string[])  [unwired: 2 in, 2 out]
                  n220 = Index Array(array=w368, index=w367) -> (element=w366:string)
                  n221 = Fract/Exp String To Number(string=w366) -> (number=w365:dbl)  [unwired: 3 in, 1 out]
                  n222 = Build Array(w365) -> (→"Rx Struct Data":dbl[])
                }
              }
            }
          }
          frame #2 {
            n223 = property on="Rx Struct Data" class="Arr (strict)"() -> ("Value"=w375:dbl[])  [unwired: 2 in, 2 out]
            n224 = property on="number" class="DigNum (strict)"() -> ("Value"=w383:i32)  [unwired: 2 in, 2 out]
            n225 = Array To Cluster(array=w375) -> (cluster=w376:T5)
            n226 = Unbundle(w376) -> ("Value[0]"=w377:dbl, "Value[1]"=w378:dbl, "Value[2]"=w379:dbl, "Value[3]"=w380:dbl, "Value[4]"=w381:dbl, "Value[5]"=w382:dbl)
            n227 = Bundle("Value[0]"=w377, "Value[1]"=w378, "Value[2]"=w379, "Value[3]"=w380, "Value[4]"=w381, "Value[5]"=w382, "Value"=w383) -> (→"Rx Data":T6)  [unwired: 1 in]
          }
        }
        n228 = IP To String(1:TRUE ("dot notation? (F)"), 2:w115) -> (0:→"IP":string)
        n229 = property on="OK Button" class="Bool (strict)"("Val(Sgnl)"=w99) -> ()  [unwired: 2 in, 2 out]
      }
    }
    n230 = case shown="True" "Export" {
      frame False {
      }
      frame True {
        n231 = flat-sequence {
          tunnel: [w30] -> w27
          tunnel: [w29] -> w26
          tunnel: [w28] -> w25
          tunnel: w27 -> [w85]
          tunnel: w26 -> [w84]
          tunnel: w25 -> [w83]
          frame #0 {
            n232 = stacked-sequence {
              tunnel: [_ w38 _ _] -> w30
              tunnel: [_ _ w45 _] -> w29
              tunnel: [_ _ _ w54] -> w28
              frame #0 {
                w33 = T3."Disabled and Grayed Out" ("Disabled")
                n233 = property on="EXCEL_STATUS" class="Str"("Text.TextColor"=u32 14417920 ("Text.Text Colors:Text Color")) -> ()  [unwired: 2 in, 2 out]
                n234 = property on="EXCEL_STATUS" class="Str"("Text.FontBold"=TRUE ("Text.Font:Bold")) -> ()  [unwired: 2 in, 2 out]
                n235 = property on="EXCEL_STATUS" class="Str"("Text.Colors"=T4 {"Foreground Color"=16777216, "Background Color"=16777216}) -> ()  [unwired: 2 in, 2 out]
                n236 = property on="EXCEL_STATUS" class="Str"("Visible"=TRUE) -> ()  [unwired: 2 in, 2 out]
                n237 = property on="EXCEL_STATUS" class="Str"("Text.BGColor"=u32 16777216 ("Text.Text Colors:BG Color")) -> ()  [unwired: 2 in, 2 out]
                n238 = property on="Export" class="Bool"("DisabledEnum"=w33) -> ()  [unwired: 2 in, 2 out]
                n239 = property on="OK Button" class="Bool (strict)"("DisabledEnum"=w33) -> ()  [unwired: 2 in, 2 out]
                n240 = property on="EXCEL_STATUS" class="Str"("Blinking"=TRUE) -> ()  [unwired: 2 in, 2 out]
              }
              frame #1 {
                n241 = case shown="True" "Tx Latency" {
                  tunnel: [cluster{"Value":i32[], "Value":u32[]} {"Value"=[], "Value"=[]} ("Cluster") w44] -> w38
                  frame False {
                  }
                  frame True {
                    n242 = property on="TxLatencyArray" class="Arr (strict)"() -> ("Value"=w42:u32[])  [unwired: 2 in, 2 out]
                    n243 = property on="TxSampleArray" class="Arr (strict)"() -> ("Value"=w41:dbl[])  [unwired: 2 in, 2 out]
                    n244 = call "StoreArrays_V2.vi"("Numeric"=0.0, "Value"=w42, "Value 2"=w41) -> ("Cluster"=w44:cluster{"Value 2":i32[], "Value":u32[]})  [unwired: 8 in]
                  }
                }
              }
              frame #2 {
                n245 = case shown="True" "Rx Latency" {
                  tunnel: [cluster{"Value":i32[], "Value":u32[]} {"Value"=[], "Value"=[]} ("Cluster") w48] -> w45
                  frame False {
                  }
                  frame True {
                    n246 = flat-sequence {
                      tunnel: [w53] -> w48
                      frame #0 {
                        n247 = Wait (ms)(milliseconds to wait=u32 2000) -> ()  [unwired: 1 out]
                      }
                      frame #1 {
                        n248 = property on="RxLatencyArray" class="Arr (strict)"() -> ("Value"=w51:dbl[])  [unwired: 2 in, 2 out]
                        n249 = property on="RxSampleArray" class="Arr (strict)"() -> ("Value"=w50:dbl[])  [unwired: 2 in, 2 out]
                        n250 = call "StoreArrays_V2.vi"("Numeric"=1.0, "Value"=w51, "Value 2"=w50) -> ("Cluster"=w53:cluster{"Value 2":i32[], "Value":u32[]})  [unwired: 8 in]
                      }
                    }
                  }
                }
              }
              frame #3 {
                n251 = case shown="True" "Total Latency" {
                  tunnel: [cluster{"Value 2":i32[], "Value":u32[]} {"Value 2"=[], "Value"=[]} ("Cluster") w57] -> w54
                  frame False {
                  }
                  frame True {
                    n252 = flat-sequence {
                      tunnel: [w78] -> w57
                      frame #0 {
                        n253 = Wait (ms)(milliseconds to wait=u32 2000) -> ()  [unwired: 1 out]
                      }
                      frame #1 {
                        n254 = property on="RxLatencyArray" class="Arr (strict)"() -> ("Value"=w60:dbl[])  [unwired: 2 in, 2 out]
                        n255 = Array Size(array=w60) -> (size(s)=w59:i32)
                        n256 = for {
                          N: w59 -> [_]
                          i -> [w61]
                          n257 = Equal To 0?(x=w61) -> (x = 0?=w62:bool)
                          n258 = case shown="True" w62 {
                            tunnel: w61 -> [w63 w75]
                            frame False {
                              n259 = property on="TxLatencyArray" class="Arr (strict)"() -> ("Value"=w67:u32[])  [unwired: 2 in, 2 out]
                              n260 = property on="RxLatencyArray" class="Arr (strict)"() -> ("Value"=w68:dbl[])  [unwired: 2 in, 2 out]
                              n261 = property on="TotalLatencyArray" class="Arr (strict)"() -> ("Value"=w70:dbl[])  [unwired: 2 in, 2 out]
                              n262 = Index Array(array=w68, index=w63) -> (element=w66:dbl)
                              n263 = Index Array(array=w67, index=w63) -> (element=w65:u32)
                              n264 = Add(x=w66, y=w65) -> (x+y=w64:dbl)
                              n265 = Insert Into Array(array=w70, index=w63, new element=w64) -> (w69:dbl[])
                              n266 = property on="TotalLatencyArray" class="Arr (strict)"("Val(Sgnl)"=w69) -> ()  [unwired: 2 in, 2 out]
                            }
                            frame True {
                              n267 = property on="TxLatencyArray" class="Arr (strict)"() -> ("Value"=w77:u32[])  [unwired: 2 in, 2 out]
                              n268 = property on="RxLatencyArray" class="Arr (strict)"() -> ("Value"=w76:dbl[])  [unwired: 2 in, 2 out]
                              n269 = Index Array(array=w76, index=w75) -> (element=w73:dbl)
                              n270 = Index Array(array=w77, index=w75) -> (element=w72:u32)
                              n271 = Add(x=w73, y=w72) -> (x+y=w74:dbl)
                              n272 = Build Array(w74) -> (→"TotalLatencyArray":dbl[])
                            }
                          }
                        }
                      }
                      frame #2 {
                        n273 = property on="TotalLatencyArray" class="Arr (strict)"() -> ("Value"=w80:dbl[])  [unwired: 2 in, 2 out]
                        n274 = property on="RxSampleArray" class="Arr (strict)"() -> ("Value"=w79:dbl[])  [unwired: 2 in, 2 out]
                        n275 = call "StoreArrays_V2.vi"("Numeric"=2.0, "Value"=w80, "Value 2"=w79) -> ("Cluster"=w78:cluster{"Value 2":i32[], "Value":u32[]})  [unwired: 8 in]
                      }
                    }
                  }
                }
              }
            }
          }
          frame #1 {
            n276 = Build Array(w85, w84, w83) -> (→"Latency Data":cluster{"Value 2":i32[], "Value":u32[]}[])
          }
          frame #2 {
            w86 = T3."Enabled" ("Disabled")
            n277 = property on="EXCEL_STATUS" class="Str"("Visible"=FALSE) -> ()  [unwired: 2 in, 2 out]
            n278 = property on="Export" class="Bool"("DisabledEnum"=w86) -> ()  [unwired: 2 in, 2 out]
            n279 = property on="OK Button" class="Bool (strict)"("DisabledEnum"=w86) -> ()  [unwired: 2 in, 2 out]
          }
        }
      }
    }
    "stringBuffer" <- ""
  }
